vi "file list -- accumulate V5.vi"(11 "tfolder path":path=path "/snowfall/Users/arcadi/Desktop/Ultrasound/Experiment/YBCO_4/Round1/Sweep12/June_2011/062511/221.16400K_300_3100_001_062511.dat") -> (0 "timestamp":dbl[](array[numeric]), 2 "sweep file name array":T1[](array[typedef]), 3 "temperatures":dbl[](array[numeric]))   [LabVIEW 2020]
uses:
  sweep file name.ctl
  file -- list data files in mmddyy folder -- V2.vi
  array - sorted inexes.vi
  find all matching strings in the list.vi
  Split file name.vi
  file -- scan filename logic -- V1.vi
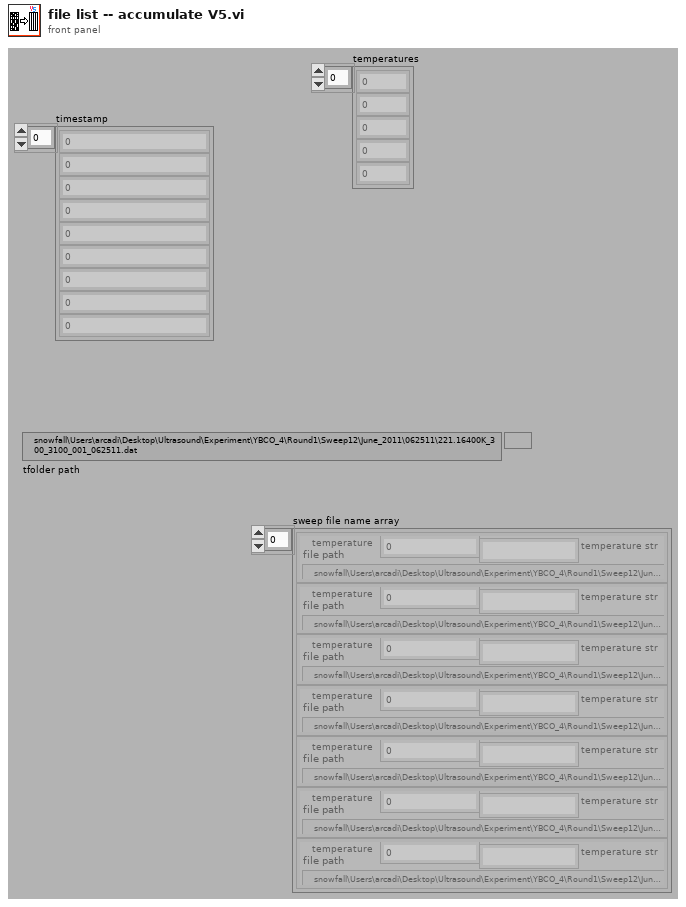
[diagram p1: front panel]
types:
  T1 = typedef "sweep file name.ctl" = cluster{"temperature":dbl, "temperature str":string, "file path":path, "last mod":timestamp, "file name str":string, "mod time(min)":dbl, "file format":enum16{"", "ascii", "binary"}, "power(V)":dbl, "Magn Field(T) ":dbl}
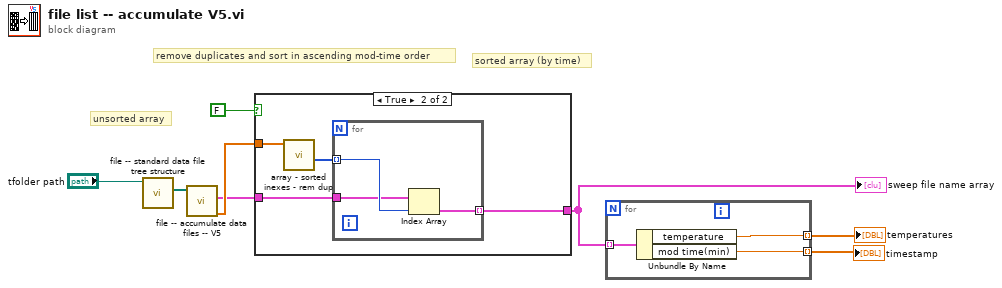
[diagram p0: block diagram]
diagram:
  # "sorted array (by time)"
  # "unsorted array"
  # "remove duplicates and sort in ascending mod-time order"
  n1 = call "file -- standard data file tree structure.vi"("folder path"="tfolder path") -> ("Array"=w7:path[])  [unwired: 10 in]
  n2 = call "file -- accumulate data files -- V5.vi"("list of <mmddyy> folders"=w7) -> ("timestamp (min) array"=w6:dbl[], "sweep file name  array"=w5:T1[])  [unwired: 9 in]
  n3 = case shown="True" FALSE {
    tunnel: w6 -> [_ w13]
    tunnel: w5 -> [w9 w11]
    tunnel: [w9 w10] -> w4
    frame False {
    }
    frame True {
      n4 = call "array - sorted inexes - rem dup.vi"("x"=w13) -> ("index array"=w12:i32[])  [unwired: 9 in, 1 out]
      n5 = for {
        tunnel: w12 -> [w15] mode=indexing
        tunnel: [w16] -> w10 mode=indexing
        tunnel: w11 -> [w14]
        n6 = Index Array(array=w14, index=w15) -> (element=w16:T1)
      }
    }
  }
  "sweep file name array" <- w4
  n7 = for {
    tunnel: w4 -> [w19] mode=indexing
    tunnel: [w18] -> w2 mode=indexing
    tunnel: [w17] -> w1 mode=indexing
    n8 = Unbundle By Name(w19) -> ("temperature"=w18:dbl, "mod time(min)"=w17:dbl)
  }
  "temperatures" <- w2
  "timestamp" <- w1
